vi "controlContinuousBkwd.vi"(7 "Set":bool, 8 "error in":errorcluster, 9 "continous BWD in":bool=TRUE, 10 "axis in":u8, 11 "connection ID":refnum<k5>) -> (0 "error out":errorcluster, 1 "continous BWD out":bool=TRUE, 2 "axis out":u8, 3 "connection ID":refnum<k5>)   [LabVIEW 2016, in "AMC_VIs.lvlib"]
doc: "Start/Stops the continuous backward move (boolean 'set') or retrieves the information, if backward continuous movement is currently happening (boolean 'get')."
uses:
  AMC_VIs.lvlib
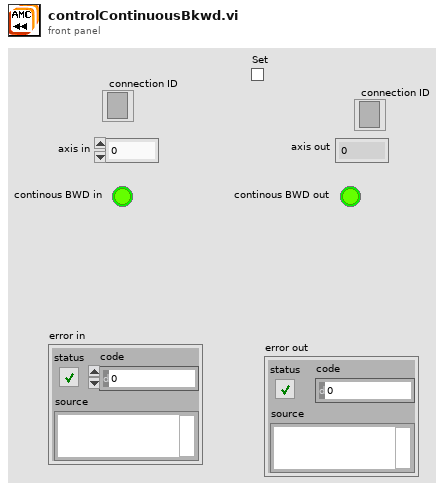
[diagram p1: front panel]
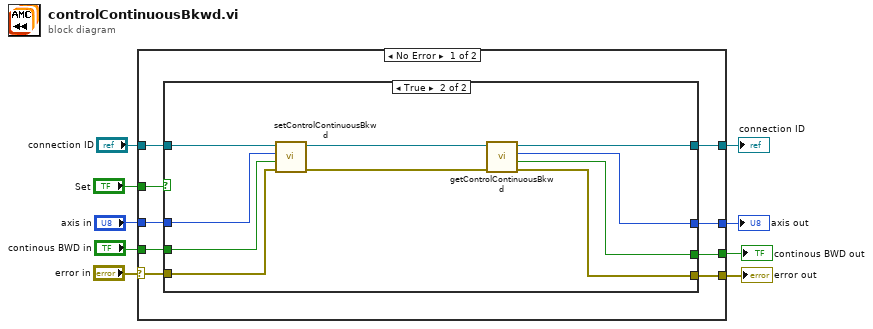
[diagram p0: block diagram]
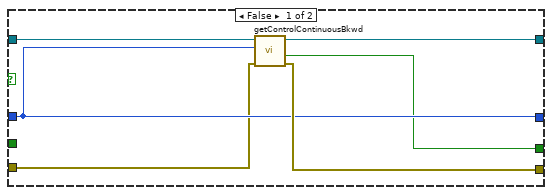
[diagram p2: hidden frame]
diagram:
  n1 = case shown="No Error" "error in" {
    selector: "error in" -> [w10 w38]
    tunnel: "axis in" -> [w16 w36]
    tunnel: [w11 w38] -> w8
    tunnel: [w13 w36] -> w7
    tunnel: "Set" -> [w17 _]
    tunnel: [w12 w37] -> w5
    tunnel: "continous BWD in" -> [w15 w37]
    tunnel: [w14 w35] -> w3
    tunnel: "connection ID" -> [w18 w35]
    frame No Error {
      n2 = case shown="True" w17 {
        tunnel: [w23 w30] -> w14
        tunnel: w18 -> [w24 w34]
        tunnel: w16 -> [w21 w32]
        tunnel: [w21 w26] -> w13
        tunnel: [w20 w27] -> w12
        tunnel: [w22 w28] -> w11
        tunnel: w15 -> [_ w33]
        tunnel: w10 -> [w19 w25]
        frame False {
          n3 = call "getControlContinuousBkwd.vi"("error in"=w19, "axis"=w21, "connection ID"=w24) -> ("error out"=w22:errorcluster, "enabled"=w20:bool, "connection ID"=w23:refnum<k5>)  [unwired: 5 in, 1 out]
        }
        frame True {
          n4 = call "setControlContinuousBkwd.vi"("error in"=w25, "enable"=w33, "axis"=w32, "connection ID"=w34) -> ("error out"=w29:errorcluster, "connection ID"=w31:refnum<k5>)  [unwired: 5 in, 1 out]
          n5 = call "getControlContinuousBkwd.vi"("error in"=w29, "connection ID"=w31) -> ("error out"=w28:errorcluster, "enabled"=w27:bool, "axis_out"=w26:i32, "connection ID"=w30:refnum<k5>)  [unwired: 6 in]
        }
      }
    }
    frame Error {
    }
  }
  "error out" <- w8
  "axis out" <- w7
  "continous BWD out" <- w5
  "connection ID" <- w3
